vi "RandomCoordinate.vi"() -> (3 "Coordinate":T1)   [LabVIEW 2019, in "RT_Game.lvlib" / "Game.lvclass"]
uses:
  Game.lvclass
  Coordinate.ctl
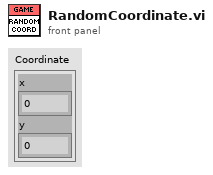
[diagram p1: front panel]
types:
  T1 = typedef "RT_Game.lvlib/Game.lvclass/Coordinate.ctl" = cluster{"x":dbl, "y":dbl}
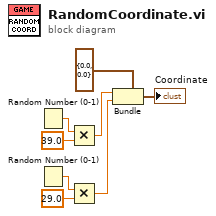
[diagram p0: block diagram]
diagram:
  n1 = Random Number (0-1)() -> (number: 0 to 1=w8:dbl)
  n2 = Random Number (0-1)() -> (number: 0 to 1=w5:dbl)
  n3 = Multiply(x=w8, y=39.0) -> (x*y=w3:dbl)
  n4 = Multiply(x=w5, y=29.0) -> (x*y=w2:dbl)
  n5 = Bundle(cluster=T1 {"x"=0.0, "y"=0.0} ("Coordinate"), "x"=w3, "y"=w2) -> (→"Coordinate":T1)
